vi "Close.vi"(8 "error in (no error)":errorcluster, 11 "EventLogHandle in":refnum<class "EventLogHandle.lvclass">) -> (0 "error out":errorcluster)   [LabVIEW 2024, in "EventLogHandle.lvclass"]
uses:
  EventLogHandle.lvclass
  EventLogHandle.lvclass/EventLogHandle.ctl
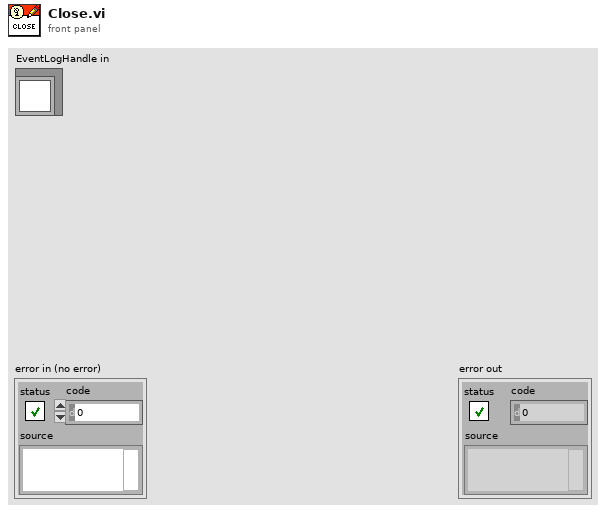
[diagram p1: front panel]
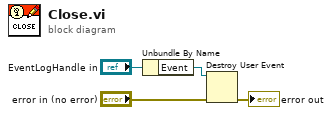
[diagram p0: block diagram]
diagram:
  n1 = Unbundle By Name("EventLogHandle in") -> ("Event"=w3:refnum<user-event>)
  n2 = Destroy User Event(user event=w3, error in="error in (no error)") -> (error out=→"error out":errorcluster)
